vi "Get Path Loss.vi"(7 "Path":T1, 8 "error in (no error)":errorcluster, 10 "Frequency [Hz]":dbl, 11 "PathControl in":refnum<class "PathControl.lvclass">) -> (0 "error out":errorcluster, 1 "Parameter":cluster{"Name":string, "Value":string}, 2 "Insertion Loss (dB)":dbl, 3 "PathControl out":refnum<class "PathControl.lvclass">)   [LabVIEW 2020, in "PathControl.lvclass"]
uses:
  PathControl.lvclass
  Paths.ctl
  PathControl.lvclass/PathControl.ctl
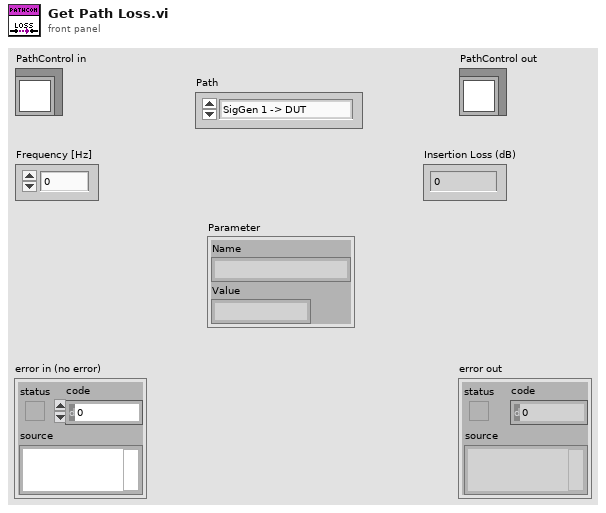
[diagram p1: front panel]
types:
  T1 = typedef "PathControl.lvclass/Paths.ctl" = enum16{"SigGen 1 -> DUT", "SigGen 2 -> DUT", "SigGen 1 -> PM 1", "SigGen 1 -> PM 2", "DUT -> SA", "DUT -> PM 2", "VSG -> DUT", "SigGen 2 -> PM 1", "SigGen 2 -> PM 2"}
  T2 = cluster{"Name":string, "Path Frequency":dbl[], "Path Loss":dbl[]}[]
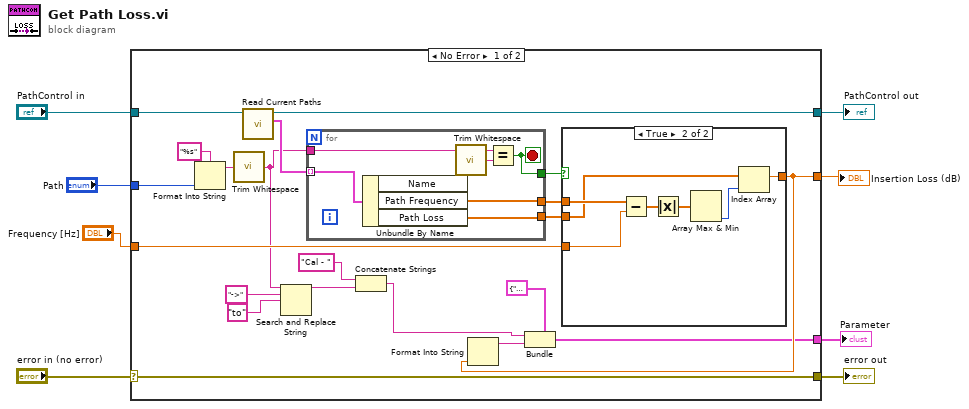
[diagram p0: block diagram]
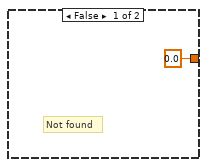
[diagram p2: hidden frame]
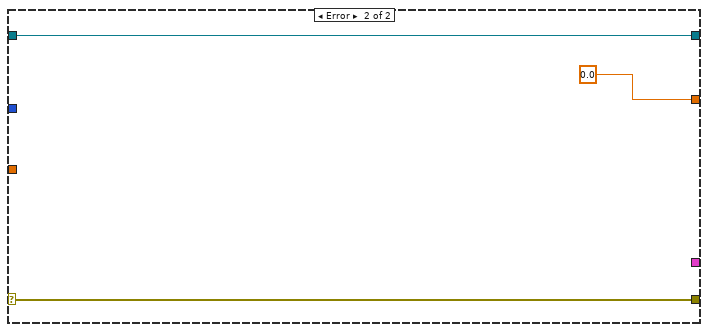
[diagram p3: hidden frame]
diagram:
  n1 = case shown="No Error" "error in (no error)" {
    selector: "error in (no error)" -> [w29 w47]
    tunnel: [w29 w47] -> w7
    tunnel: [w27 w46] -> w5
    tunnel: "PathControl in" -> [w28 w46]
    tunnel: [w17 0.0] -> w4
    tunnel: "Path" -> [w24 _]
    tunnel: "Frequency [Hz]" -> [w21 _]
    tunnel: [w16 _] -> w1
    frame No Error {
      n2 = Format Into String(format string="%s", w24) -> (resulting string=w23:string)  [unwired: 2 in, 1 out]
      n3 = call <vilib>:"Trim Whitespace.vi"("string"=w23) -> ("trimmed string"=w12:string)  [unwired: 1 in]
      n4 = call "Read Current Paths.vi"("PathControl in"=w28) -> ("Current Paths"=w26:T2, "PathControl out"=w27:refnum<class "PathControl.lvclass">)  [unwired: 9 in]
      n5 = Search and Replace String(input string=w12, search string="->", replace string="to" ("replace string (\"\")")) -> (result string=w11:string)  [unwired: 5 in, 3 out]
      n6 = for {
        tunnel: w26 -> [w44] mode=indexing
        tunnel: w12 -> [w42]
        tunnel: [w41] -> w22
        tunnel: [w40] -> w20
        tunnel: [w38] -> w19
        stop <- w38 stop-if-true
        n7 = Unbundle By Name(w44) -> ("Name"=w43:string, "Path Frequency"=w41:dbl[], "Path Loss"=w40:dbl[])
        n8 = call <vilib>:"Trim Whitespace.vi"("string"=w43) -> ("trimmed string"=w39:string)  [unwired: 1 in]
        n9 = Equal?(x=w42, y=w39) -> (x = y?=w38:bool)
      }
      n10 = Concatenate Strings("Cal - " ("string"), w11) -> (w10:string)
      n11 = case shown="True" w19 {
        tunnel: w22 -> [_ w37]
        tunnel: w21 -> [_ w36]
        tunnel: w20 -> [_ w32]
        tunnel: [0.0 ("Numeric Control") w31] -> w17
        frame False {
          # "Not found"
        }
        frame True {
          n12 = Subtract(x=w37, y=w36) -> (x-y=w35:dbl[])
          n13 = Absolute Value(x=w35) -> (abs(x)=w34:dbl[])
          n14 = Array Max & Min(array=w34) -> (min index (indices)=w33:i32)  [unwired: 3 out]
          n15 = Index Array(array=w32, index=w33) -> (element=w31:dbl)
        }
      }
      n16 = Format Into String(w17) -> (resulting string=w15:string)  [unwired: 3 in, 1 out]
      n17 = Bundle(cluster=cluster{"Name":string, "Value":string} {"Name"="", "Value"=""} ("Change"), "Name"=w10, "Value"=w15) -> (w16:cluster{"Name":string, "Value":string})
    }
    frame Error {
    }
  }
  "error out" <- w7
  "PathControl out" <- w5
  "Insertion Loss (dB)" <- w4
  "Parameter" <- w1
